vi "Boolean String to Bool.vi"(1 "boolean string":string(combo)="FALSE") -> (0 "true?":bool)   [LabVIEW 2017]
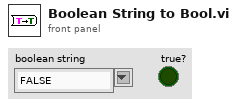
[diagram p1: front panel]
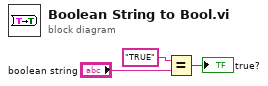
[diagram p0: block diagram]
diagram:
  n1 = Equal?(x="TRUE", y="boolean string") -> (x = y?=→"true?":bool)
